vi "KINECT_Init_Calibrate.vi"(10 "Muscle Tolerance":dbl=0.05, 11 "Skeleton Vertices":cluster{"x":sgl, "y":sgl, "z":sgl}[](array[cluster])) -> (2 "Go to Calibrate":bool)   [LabVIEW 2011]
uses:
  <vilib>/addons/Kinect/Skeleton Vertex Index.ctl
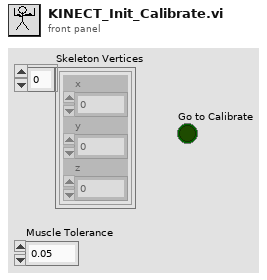
[diagram p1: front panel]
types:
  T1 = typedef "Skeleton Vertex Index.ctl" = i32
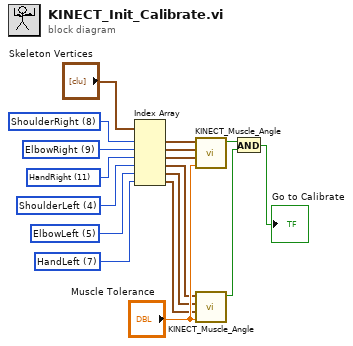
[diagram p0: block diagram]
diagram:
  w11 = T1 7 items=["HipCenter", "Spine", "ShoulderCenter", "Head", "ShoulderLeft", "ElbowLeft", "WristLeft", "HandLeft", "ShoulderRight", "ElbowRight", "WristRight", "HandRight", "HipLeft", "KneeLeft", "AnkleLeft", "FootLeft", "HipRight", "KneeRight", "AnkleRight", "FootRight"] ("Skeleton Joints")
  w10 = T1 5 items=["HipCenter", "Spine", "ShoulderCenter", "Head", "ShoulderLeft", "ElbowLeft", "WristLeft", "HandLeft", "ShoulderRight", "ElbowRight", "WristRight", "HandRight", "HipLeft", "KneeLeft", "AnkleLeft", "FootLeft", "HipRight", "KneeRight", "AnkleRight", "FootRight"] ("Skeleton Joints")
  w9 = T1 4 items=["HipCenter", "Spine", "ShoulderCenter", "Head", "ShoulderLeft", "ElbowLeft", "WristLeft", "HandLeft", "ShoulderRight", "ElbowRight", "WristRight", "HandRight", "HipLeft", "KneeLeft", "AnkleLeft", "FootLeft", "HipRight", "KneeRight", "AnkleRight", "FootRight"] ("Skeleton Joints")
  w3 = T1 9 items=["HipCenter", "Spine", "ShoulderCenter", "Head", "ShoulderLeft", "ElbowLeft", "WristLeft", "HandLeft", "ShoulderRight", "ElbowRight", "WristRight", "HandRight", "HipLeft", "KneeLeft", "AnkleLeft", "FootLeft", "HipRight", "KneeRight", "AnkleRight", "FootRight"] ("Skeleton Joints")
  w4 = T1 11 items=["HipCenter", "Spine", "ShoulderCenter", "Head", "ShoulderLeft", "ElbowLeft", "WristLeft", "HandLeft", "ShoulderRight", "ElbowRight", "WristRight", "HandRight", "HipLeft", "KneeLeft", "AnkleLeft", "FootLeft", "HipRight", "KneeRight", "AnkleRight", "FootRight"] ("Skeleton Joints")
  w2 = T1 8 items=["HipCenter", "Spine", "ShoulderCenter", "Head", "ShoulderLeft", "ElbowLeft", "WristLeft", "HandLeft", "ShoulderRight", "ElbowRight", "WristRight", "HandRight", "HipLeft", "KneeLeft", "AnkleLeft", "FootLeft", "HipRight", "KneeRight", "AnkleRight", "FootRight"] ("Skeleton Joints")
  n1 = Index Array(array="Skeleton Vertices", index #1=w2, index #2=w3, index #3=w4, index #4=w9, index #5=w10, index #6=w11) -> (element #1=w5:cluster{"x":sgl, "y":sgl, "z":sgl}, element #2=w6:cluster{"x":sgl, "y":sgl, "z":sgl}, element #3=w7:cluster{"x":sgl, "y":sgl, "z":sgl}, element #4=w12:cluster{"x":sgl, "y":sgl, "z":sgl}, element #5=w13:cluster{"x":sgl, "y":sgl, "z":sgl}, element #6=w14:cluster{"x":sgl, "y":sgl, "z":sgl})
  n2 = call "KINECT_Muscle_Angle.vi"("Muscle Tolerance"="Muscle Tolerance", "Hand"=w7, "Elbow"=w6, "Shoulder"=w5) -> ("Go to Calibrate"=w17:bool)  [unwired: 7 in]
  n3 = call "KINECT_Muscle_Angle.vi"("Muscle Tolerance"="Muscle Tolerance", "Hand"=w14, "Elbow"=w13, "Shoulder"=w12) -> ("Go to Calibrate"=w16:bool)  [unwired: 7 in]
  n4 = And(x=w17, y=w16) -> (x .and. y?=→"Go to Calibrate":bool)
